vi "GetDescendantType.vi"(8 "error in (no error)":errorcluster, 10 "To Object":refnum<class>, 11 "From Object":refnum<class>) -> (0 "error out":errorcluster, 1 "Descent Type":T1=enum."less specific", 2 "To Object (dup)":refnum<class>, 3 "From Object (dup)":refnum<class>)   [LabVIEW 2020, in "BlueSerialization.lvlib" / "BlueSerializer.lvclass"]
uses:
  BlueSerializer.lvclass
  ClassNameSummary.ctl
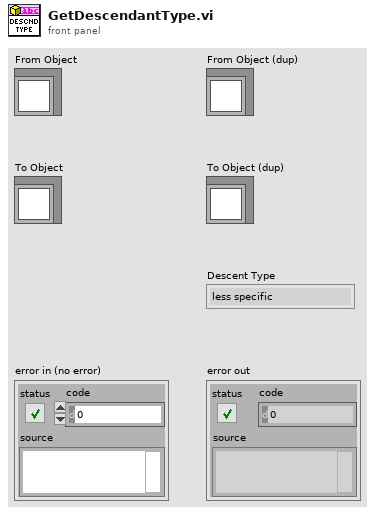
[diagram p1: front panel]
types:
  T1 = typedef "BlueSerialization.lvlib/BlueSerializer.lvclass/ClassNameSummary.ctl" = enum16{"sibling", "more specific", "less specific", "same"}
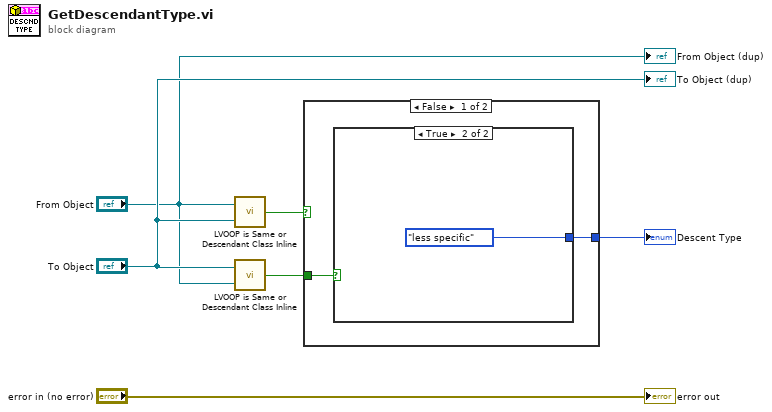
[diagram p0: block diagram]
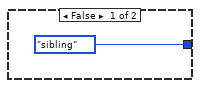
[diagram p2: hidden frame]
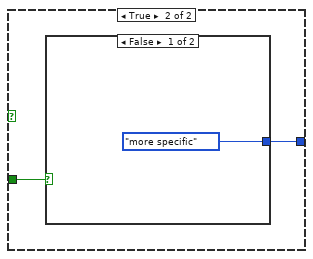
[diagram p3: hidden frame]
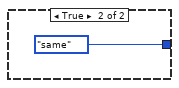
[diagram p4: hidden frame]
diagram:
  n1 = call "LVOOP is Same or Descendant Class Inline.vi"("Possible Descendant Object"="To Object", "Object"="From Object") -> ("Is Same Class or Descendant?"=w4:bool)
  n2 = call "LVOOP is Same or Descendant Class Inline.vi"("Possible Descendant Object"="From Object", "Object"="To Object") -> ("Is Same Class or Descendant?"=w1:bool)
  n3 = case shown="False" w4 {
    tunnel: w1 -> [w8 w12]
    tunnel: [w7 w11] -> w6
    frame False {
      n4 = case shown="True" w8 {
        tunnel: [ClassNameSummary."sibling" ("Enum") ClassNameSummary."less specific" ("Enum")] -> w7
        frame False {
        }
        frame True {
        }
      }
    }
    frame True {
      n5 = case shown="False" w12 {
        tunnel: [ClassNameSummary."more specific" ("Enum") ClassNameSummary."same" ("Enum")] -> w11
        frame False {
        }
        frame True {
        }
      }
    }
  }
  "Descent Type" <- w6
  "error out" <- "error in (no error)"
  "From Object (dup)" <- "From Object"
  "To Object (dup)" <- "To Object"
